vi "Modbus to String.vi"(10 "Registers":u16[](array[numeric])) -> (2 "String":string)   [LabVIEW 2024, in "Bronkhorst Flexi-Flow ModbusTCP API.lvlib"]
uses:
  Bronkhorst Flexi-Flow ModbusTCP API.lvlib
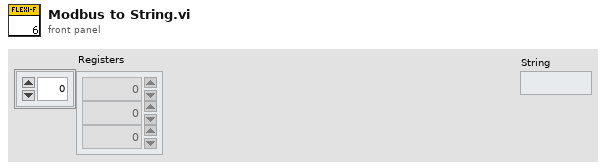
[diagram p1: front panel]
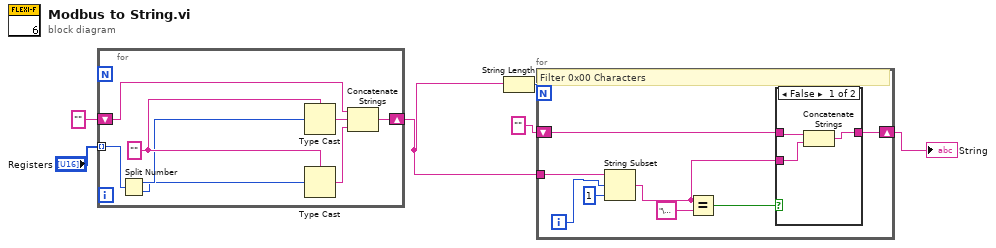
[diagram p0: block diagram]
diagram:
  n1 = for {
    tunnel: "Registers" -> [w14] mode=indexing
    shift-right: [w10] -> w2
    shift-left: "" -> [w9]
    w12 = "" ("type")
    n2 = Split Number(x=w14) -> (hi(x)=w8:u8, lo(x)=w7:u8)
    n3 = Type Cast(type=w12, x=w8) -> (*(type *) &x=w13:string)
    n4 = Type Cast(type=w12, x=w7) -> (*(type *) &x=w11:string)
    n5 = Concatenate Strings(w9, w13, w11) -> (w10:string)
  }
  n6 = String Length(string=w2) -> (length=w4:i32)
  n7 = for {
    N: w4 -> [_]
    shift-right: [w18] -> w1
    shift-left: "" -> [w17]
    tunnel: w2 -> [w15]
    i -> [w21]
    # "Filter 0x00 Characters"
    n8 = String Subset(string=w15, offset (0)=w21, length (rest)=1 ("length (rest)")) -> (substring=w16:string)
    n9 = Equal?(x=w16, y="\u0000") -> (x = y?=w19:bool)
    n10 = case shown="False" w19 {
      tunnel: [w23 w26] -> w18
      tunnel: w17 -> [w25 w26]
      tunnel: w16 -> [w24 _]
      frame False {
        n11 = Concatenate Strings(w25, w24) -> (w23:string)
      }
      frame True {
      }
    }
  }
  "String" <- w1
